vi "Read Datalog File.vi"() -> ()   [LabVIEW 2023]
doc: "Opens the datalog file created by the Write Datalog File VI and reads one record at a time from the file. Each record is a cluster containing an ID string and an array of numbers."
uses:
  support/Datalog Record.ctl
panel:
  in  "Desired Record Index":i64 min=0 max=9 step=1
  in  "Stop":bool
  out "Record Data":dbl[](graph)
  out "Record ID":string
  # "Overview: Demonstrates the use of the Datalog functions to read data from a datalog file.\nInstructions:\n1. Make sure you have already run Write Datalog File.vi.\n2. Run this VI. The data at the Desired Record Index will be displayed in the Record Data and Record ID indicators.\n3. Change the Desired Record Index value to see different records stored in the datalog file.\n4. Click Stop to stop the VI.\n5. Delete the datalog file (located at [LabVIEW Data]\\Example Datalog File.dat) when you are done."
  # "Note: Since the Write Datalog File VI writes 10 records to the datalog file, this numeric control is configured to only allow values between 0 and 9. Right-click a numeric control and select Data Entry to configure upper and lower data entry limits on numeric controls."
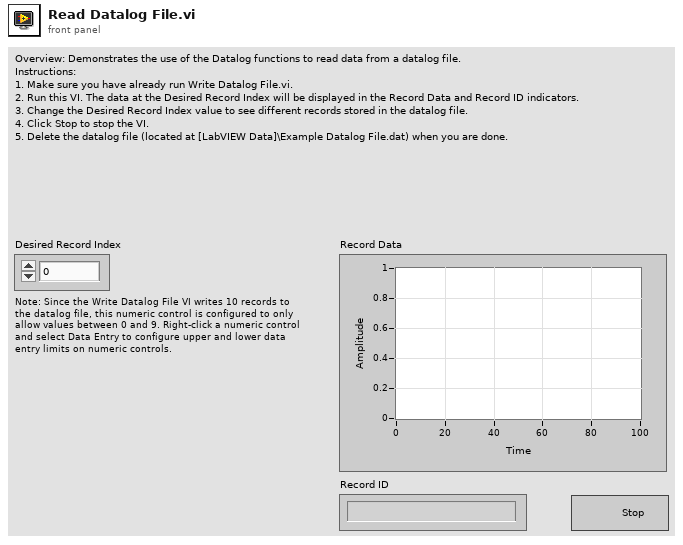
[diagram p1: front panel]
types:
  T1 = typedef "Datalog Record.ctl" = cluster{"Record ID String":string, "Numeric Data":dbl[]}
  T2 = enum16{"open", "replace", "create", "open or create", "replace or create", "replace or create with confirmation"}
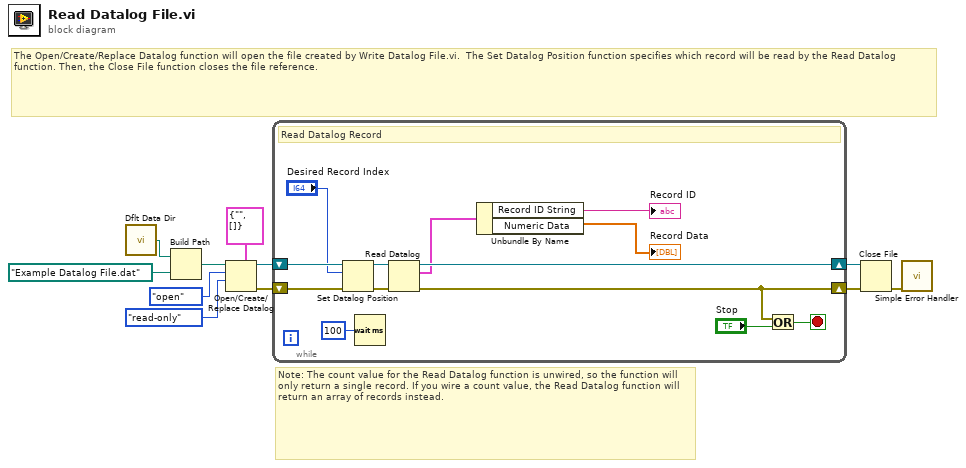
[diagram p0: block diagram]
diagram:
  # "Note: The count value for the Read Datalog function is unwired, so the function will only return a single record. If you wire a count value, the Read Datalog function will return an array of records instead."
  # "The Open/Create/Replace Datalog function will open the file created by Write Datalog File.vi.  The Set Datalog Position function specifies which record will be read by the Read Datalog function. Then, the Close File function closes the file reference."
  n1 = call <vilib>:"Dflt Data Dir.vi"() -> ("App:Default Data Directory"=w6:path)
  n2 = Build Path(base path=w6, name or relative path=path "Example Datalog File.dat" ("default name")) -> (appended path=w4:path)
  n3 = Open/Create/Replace Datalog(5:T1 {"Record ID String"="", "Numeric Data"=[]} ("Datalog Record"), 9:enum16{"read/write", "read-only", "write-only"}."read-only" ("access (0:read/write)"), 10:T2."open" ("operation (0:open)"), 11:w4) -> (0:w3:errorcluster, 3:w2:refnum<k1>)  [unwired: 1 in, 2 out]
  n4 = while {
    shift-right: [w24] -> w11
    shift-left: w2 -> [w15]
    shift-right: [w19] -> w10
    shift-left: w3 -> [w20]
    stop <- w17 stop-if-true
    # "Read Datalog Record"
    n5 = Set Datalog Position(4:w20, 6:"Desired Record Index", 7:w15) -> (0:w16:errorcluster, 3:w14:refnum<k1>)  [unwired: 1 in]
    n6 = Wait (ms)(milliseconds to wait=u32 100) -> ()  [unwired: 1 out]
    n7 = Read Datalog(4:w16, 7:w14) -> (0:w19:errorcluster, 2:w23:T1, 3:w24:refnum<k1>)  [unwired: 1 out]
    n8 = Unbundle By Name(w23) -> ("Record ID String"=→"Record ID":string, "Numeric Data"=→"Record Data":dbl[])
    n9 = Or(x=w19, y="Stop") -> (x .or. y?=w17:bool)
  }
  n10 = Close File(refnum=w11, error in=w10) -> (error out=w1:errorcluster)  [unwired: 1 out]
  n11 = call <vilib>:"Simple Error Handler.vi"("error in (no error)"=w1) -> ()  [unwired: 4 in, 5 out]
